vi "ChangeYear.vi"(8 "error in (no error)":errorcluster, 10 "Year":i32, 11 "Calendar in":refnum<class "Calendar.lvclass">) -> (0 "error out":errorcluster, 3 "Calendar (dup)":refnum<class "Calendar.lvclass">)   [LabVIEW 2015, in "Calendar.lvclass"]
uses:
  Calendar.lvclass
  Calendar.lvclass/Calendar.ctl
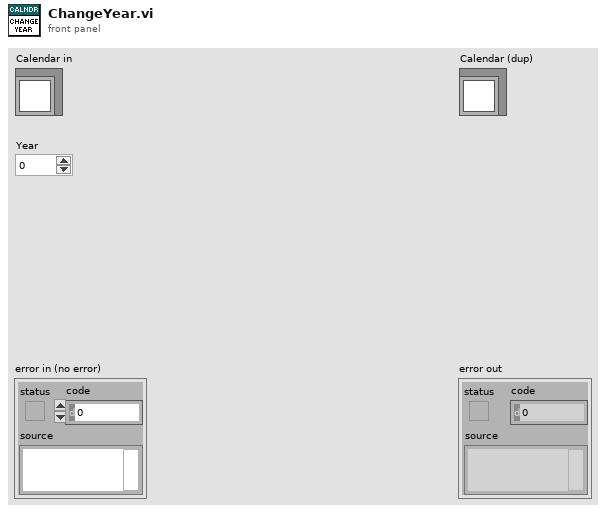
[diagram p1: front panel]
types:
  T1 = typedef "Calendar.lvclass/State Data.ctl" = cluster{"Current Date":timestamp, "First Day of Week":T2, "Color":cluster{"Selector Background":u32, "Selector Text":u32, "Days of Week Background":u32, "Days of Week Text":u32, "Calendar Background":u32, "Calendar Text":u32, "Calendar Selection Background":u32, "Calendar Selection Text":u32}, "Visible":cluster{"Today Selector Visible":bool, "Month-Year Selector Visible":bool}}
  T2 = typedef "Calendar.lvclass/DaysOfWeek.ctl" = enum16{"Sunday", "Monday", "Tuesday", "Wednesday", "Thursday", "Friday", "Saturday"}
  T3 = typedef "LVDateTimeRec.ctl" = cluster{"fractional second":dbl, "second":i32, "minute":i32, "hour":i32, "day of month":i32, "month":i32, "year":i32, "day of week":i32, "day of year":i32, "DST":i32}
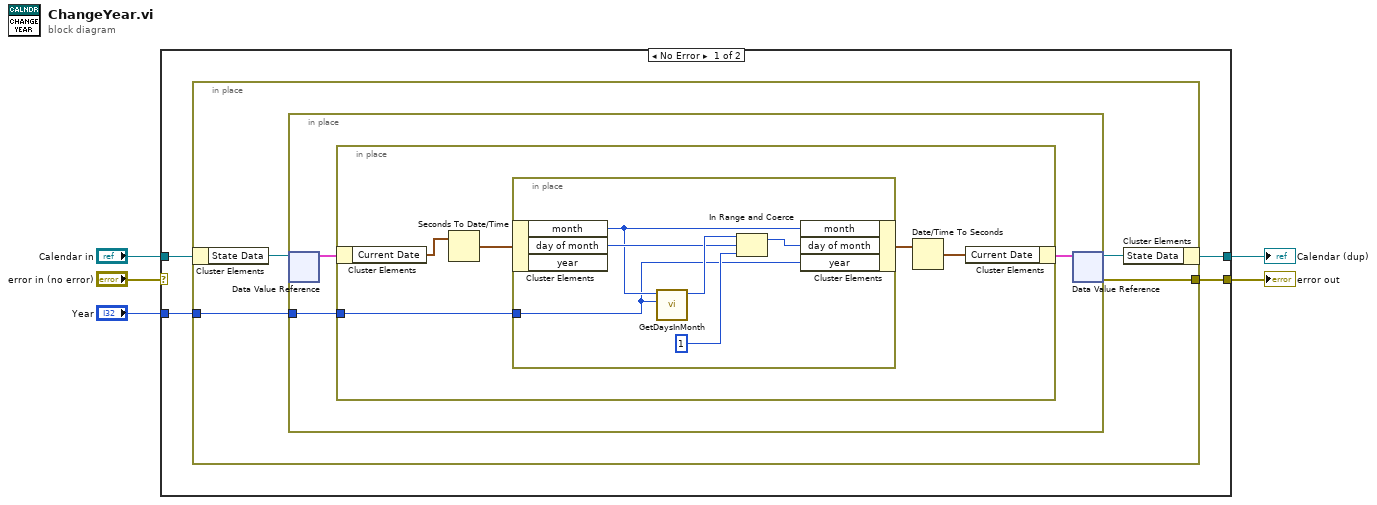
[diagram p0: block diagram]
diagram:
  n1 = case shown="No Error" "error in (no error)" {
    selector: "error in (no error)" -> [_ w29]
    tunnel: [w6 w29] -> w4
    tunnel: [w8 w28] -> w2
    tunnel: "Calendar in" -> [w9 w28]
    tunnel: "Year" -> [w7 _]
    frame No Error {
      n2 = in-place {
        in-place-border: w7 -> [w11]
        in-place-border: [w10] -> w6
        n3 = in-place-cluster #1(w9) -> ("State Data"=w13:refnum<data-value>)
        n4 = in-place {
          in-place-border: w11 -> [w14]
          n5 = in-place-dvr #2(w13) -> (w16:T1)  [unwired: 1 out]
          n6 = in-place {
            in-place-border: w14 -> [w18]
            n7 = in-place-cluster #3(w16) -> ("Current Date"=w21:timestamp)
            n8 = Seconds To Date/Time(time stamp (now)=w21) -> (date time rec=w17:T3)  [unwired: 1 in]
            n9 = in-place {
              in-place-border: w18 -> [w22]
              n10 = in-place-cluster #4(w17) -> ("month"=w23:i32, "day of month"=w24:i32)  [unwired: 1 out]
              n11 = call "GetDaysInMonth.vi"("Year"=w22, "Month"=w23) -> ("Number of Days in Month"=w26:i32)  [unwired: 8 in, 1 out]
              n12 = In Range and Coerce(upper limit=w26, x=w24, lower limit=1) -> (coerced(x)=w25:i32)  [unwired: 1 out]
              n13 = in-place-cluster #4("month"=w23, "day of month"=w25, "year"=w22) -> (w19:T3)
            }
            n14 = Date/Time To Seconds(2:w19) -> (0:w20:timestamp)  [unwired: 1 out]
            n15 = in-place-cluster #3("Current Date"=w20) -> (w15:T1)
          }
          n16 = in-place-dvr #2(w15) -> (w12:refnum<data-value>, w10:errorcluster)
        }
        n17 = in-place-cluster #1("State Data"=w12) -> (w8:refnum<class "Calendar.lvclass">)
      }
    }
    frame Error {
    }
  }
  "error out" <- w4
  "Calendar (dup)" <- w2
